vi "KH TURCK ETHERNETIP Init.vi"(6 "EIP_DO":T1 {"Nr" max=63; "Chan" max=63}, 7 "EIP_DI":T3={"Signal Name"=["IOL0", "IOL2", "ARFID0", "ARFID1", "BRFID2", "BRFID3", "ADXP1", "ADXP3", "ADXP4", "ADXP5", "BDXP0", "BDXP4", "BDXP5", "BDXP6"], "Description"=[], "Chan"=[], "Inv"=[], "Nr"=[1, 1, 1, 1, 2, 2, 1, 1, 1, 1, 2, 2, 2, 2], "SensorType"=[enum."TBEN-S2-4IOL", enum."TBEN-S2-4IOL", enum."TBEN-S2-2RFID-4DXP", enum."TBEN-S2-2RFID-4DXP", enum."TBEN-S2-2RFID-4DXP", enum."TBEN-S2-2RFID-4DXP", enum."TBEN-S1-8DXP", enum."TBEN-S1-8DXP", enum."TBEN-S1-8DXP", enum."TBEN-S1-8DXP", enum."TBEN-S1-8DXP", enum."TBEN-S1-8DXP", enum."TBEN-S1-8DXP", enum."TBEN-S1-8DXP"]} {"Nr" max=63; "Chan" max=63}, 8 "err in":errorcluster caption="error", 9 "TimeoutRFID":dbl=5.0 format="%#_13g", 10 "Parameter RFID Array":T4(array[cluster])=[{"NumberOfBytes0"=312, "SizeFragmentRead1"=128, "SizeFragmentRead0"=128, "SizeFragmentWrite0"=128, "SizeFragmentWrite1"=128, "NumberOfBytes1"=312}, {"NumberOfBytes0"=312, "SizeFragmentRead1"=128, "SizeFragmentRead0"=128, "SizeFragmentWrite0"=128, "SizeFragmentWrite1"=128, "NumberOfBytes1"=312}]) -> (0 "err out":errorcluster caption="error")   [LabVIEW 2021]
uses:
  KH_DAQ 17.04/Turck/KH_DAQ_TURCK_TypeDefs_Cluster DI.ctl
  KH EthernetIPConfig 17.14/KH EthernetIPConfig TypeDefs ModuleTyp.ctl
  KH_DAQ 17.04/Turck/KH_DAQ_TURCK_TypeDefs_Cluster DO.ctl
  KH TURCK ETHERNETIP TDef Enum IOL Data.ctl
  KH TURCK ETHERNETIP TDefCluster TBEN-S2-2RFID-4DXP Input Values.ctl
  KH EthernetIP 17.19/KH_EthernetIP_Globals.vi
  KH TURCK ETHERNETIP Global.vi
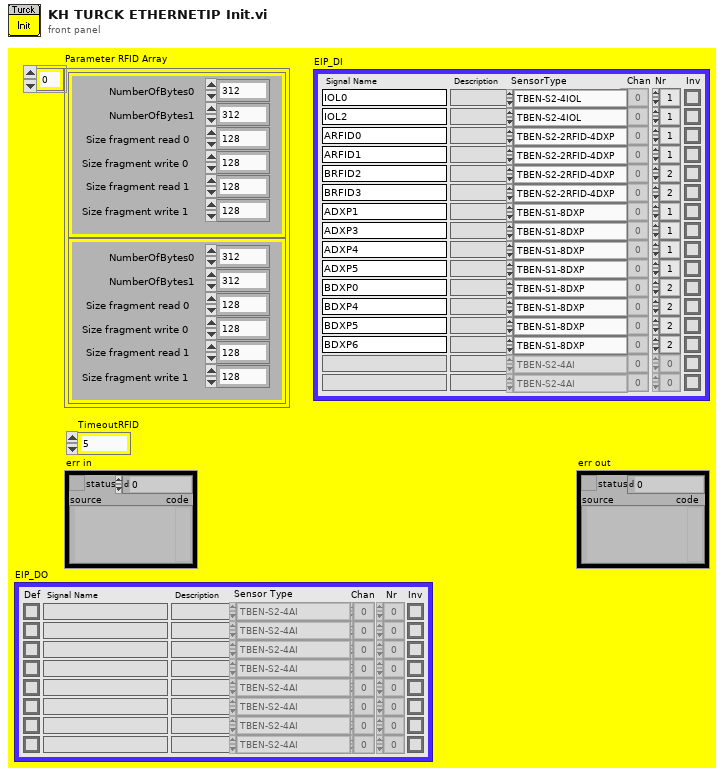
[diagram p1: front panel]
types:
  T1 = typedef "KH_DAQ_TURCK_TypeDefs_Cluster DO.ctl" = cluster{"Def":bool[], "Signal Name":string[], "Description":string[], "Chan":u16[], "Inv":bool[], "Nr":u16[], "SensorType":T2[]}
  T2 = typedef "KH EthernetIPConfig TypeDefs ModuleTyp.ctl" = enum16{"TBEN-S2-4AI", "TBEN-S1-8DXP", "TBEN-S2-2RFID-4DXP", "TBEN-S2-4AO", "TBEN-S2-4IOL"}
  T3 = typedef "KH_DAQ_TURCK_TypeDefs_Cluster DI.ctl" = cluster{"Signal Name":string[], "Description":string[], "Chan":u16[], "Inv":bool[], "Nr":u16[], "SensorType":T2[]}
  T4 = cluster{"NumberOfBytes0":i32, "SizeFragmentRead1":i32, "SizeFragmentRead0":i32, "SizeFragmentWrite0":i32, "SizeFragmentWrite1":i32, "NumberOfBytes1":i32}[]
  T5 = cluster{"Data":bool[], "Overcurrent":bool[], "Overcurrent VAUX1 Ch0-3":bool, "Overcurrent VAUX2 Ch4-7":bool, "Latch Input":bool[], "Counter value":u32, "Counter frequency (Hz)":u16, "Status":u8, "Overcurrent PWM Output 3":u8, "Overcurrent PWM Output 7":u8, "Module Diagnostics Available":bool, "INFO: ARGEE Project Running":bool, "Undervoltage V2":bool, "Undervoltage V1":bool, "Force Mode Enabled":bool}
  T6 = cluster{"Overload Ch0":bool, "Overload Ch1":bool, "Overload Ch2":bool, "Overload Ch3":bool, "Wirebreak Ch0":bool, "Wirebreak Ch1":bool, "Wirebreak Ch2":bool, "Wirebreak Ch3":bool, "Module Diagnostics Available":bool, "INFO: ARGEE Project Running":bool, "Undervoltage V2":bool, "Undervoltage V1":bool, "Internal Error":bool, "Force Mode Enabled":bool}
  T7 = cluster{"Data":i16[], "upper Limit CH0":bool, "upper Limit CH1":bool, "upper Limit CH2":bool, "upper Limit CH3":bool, "Overflow CH0":bool, "Overflow CH1":bool, "Overflow CH2":bool, "Overflow CH3":bool, "Underflow CH0":bool, "Underflow CH1":bool, "Underflow CH2":bool, "Underflow CH3":bool, "CJC Wire Break CH0":bool, "CJC Wire Break CH1":bool, "CJC Wire Break CH2":bool, "CJC Wire Break CH3":bool, "Overcurrent (RTD) CH0":bool, "Overcurrent (RTD) CH1":bool, "Overcurrent (RTD) CH2":bool, "Overcurrent (RTD) CH3":bool, "Wire Break CH0":bool, "Wire Break CH1":bool, "Wire Break CH2":bool, "Wire Break CH3":bool, "Overcurrent supply VAUX1 CH0":bool, "Overcurrent supply VAUX1 CH1":bool, "Overcurrent supply VAUX1 CH2":bool, "Overcurrent supply VAUX1 CH3":bool, "Lower limit value underrun CH0":bool, "Lower limit value underrun CH1":bool, "Lower limit value underrun CH2":bool, "Lower limit value underrun CH3":bool, "Module Diagnostics Available":bool, "INFO: ARGEE Project Running":bool, "Undervoltage Field Supply V2":bool, "Undervoltage Field Supply V1":bool, "Internal Error":bool, "Force Mode Enabled":bool}
  T8 = typedef "KH TURCK ETHERNETIP TDefCluster TBEN-S2-2RFID-4DXP Input Values.ctl" = cluster{"Station Status Word (Input Data Mapping)":cluster{"Module diagnostics avaliable":bool, "INFO: ARGEE Project Running":bool, "Undervoltage V2":bool, "Undervoltage V1":bool, "Internal Error":bool, "I/O-ASSISTANT Force Mode active":bool}, "RFID control/status 0 (Input Data Mapping)":cluster{"Tag present at r/w head":bool[], "response code":u16, "loop counter":u8, "Length":u16, "Error code":u16, "Tag counter":u16, "Data (Bytes) available":u16, "Read fragment No.":u8, "Write fragment No.":u8, "Tag present at r/w head bit":bool, "HF r/w head switched on":bool, "Continuous mode active":bool, "Antenna detuned at HF read/write head":bool, "Parameter not supported by read/write head":bool, "Error reported by read/write head":bool, "Not connected to read/write head":bool}, "RFID read data 0 (Input Data Mapping)":u8[], "RFID control/status 1 (Input Data Mapping)":cluster{"response code":u16, "Loop counter":u8, "Length":u16, "Error code":u16, "Tag counter":u16, "Data (Bytes) available":u16, "Read fragment No.":u8, "Write fragment No.":u8, "Tag present at r/w head bit":bool, "HF r/w head switched on":bool, "Continuous mode active":bool, "Antenna detuned at HF read/write head":bool, "Parameter not supported by read/write head":bool, "Error reported by read/write head":bool, "Not connected to read/write head":bool, "Tag present at r/w head":bool[]}, "RFID read data 1 (Input Data Mapping)":u8[], "RFID diagnostics (Input Data Mapping)":cluster{"Overcurrent supply VAUX1 (a)":bool, "Parameterization error (a)":bool, "Configuration via DTM active (a)":bool, "Buffer full (a)":bool, "Antenna detuned at HF read/write head (a)":bool[], "Parameter not supported by read/write head (a)":bool[], "Error reported by read/write head (a)":bool[], "Not connected to read/write head (a)":bool[], "Overcurrent supply VAUX1 (b)":bool, "Parameterization error (b)":bool, "Configuration via DTM active (b)":bool, "Buffer full (b)":bool, "Antenna detuned at HF read/write head (b)":bool[], "Parameter not supported by read/write head (b)":bool[], "Error reported by read/write head (b)":bool[], "Not connected to read/write head (b)":bool[]}, "DXP diagnostics (Input Data Mapping)":cluster{"Overcurrent VAUX2 Ch4/5":bool, "Overcurrent VAUX2 Ch6/7":bool, "Channel 4 - Output overcurrent":bool, "Channel 5 - Output overcurrent":bool, "Channel 6 - Output overcurrent":bool, "Channel 7 - Output overcurrent":bool}, "DXP (Input Data Mapping)":cluster{"Channel 4 - Input value":bool, "Channel 5 - Input value":bool, "Channel 6 - Input value":bool, "Channel 7 - Input value":bool}}
  T9 = typedef "KH TURCK ETHERNETIP TDef Enum IOL Data.ctl" = cluster{"Data_Port1":u16[], "Data_Port3":u16[], "Data_Port5":u16[], "Data_Port7":u16[], "Status":cluster{"Undervoltage Field Supply V2":bool, "Overvoltage Field Supply V1":bool, "Undervoltage Field Supply V1":bool, "Internal Error":bool, "Module Diagnostics Available":bool, "Station Configuration Changed":bool, "Overcurrent Isys":bool, "Overvoltage Field Supply V2":bool, "Force Mode Enabled":bool}, "Diagnostics":cluster{"Channel 2 - Output signal overcurrent":bool, "Channel 4 - Output signal overcurrent":bool, "Channel 6 - Output signal overcurrent":bool, "Channel 8 - Output signal overcurrent":bool, "Channel 1 - Wrong or missing device":bool, "Channel 3 - Wrong or missing device":bool, "Channel 5 - Wrong or missing device":bool, "Channel 7 - Wrong or missing device":bool, "Channel 1 - Data storage error":bool, "Channel 3 - Data storage error":bool, "Channel 5 - Data storage error":bool, "Channel 7 - Data storage error":bool, "Channel 1 - Process input data invalid":bool, "Channel 3 - Process input data invalid":bool, "Channel 5 - Process input data invalid":bool, "Channel 7 - Process input data invalid":bool, "Channel 1 - Hardware error":bool, "Channel 3 - Hardware error":bool, "Channel 5 - Hardware error":bool, "Channel 7 - Hardware error":bool, "Channel 1 - Maintenance events":bool, "Channel 3 - Maintenance events":bool, "Channel 5 - Maintenance events":bool, "Channel 7 - Maintenance events":bool, "Channel 1 - Out of spec. error":bool, "Channel 3 - Out of spec. error":bool, "Channel 5 - Out of spec. error":bool, "Channel 7 - Out of spec. error":bool, "Channel 1 - Parameterization error":bool, "Channel 3 - Parameterization error":bool, "Channel 5 - Parameterization error":bool, "Channel 1 - Overtemperature":bool, "Channel 3 - Overtemperature":bool, "Channel 5 - Overtemperature":bool, "Channel 7 - Overtemperature":bool, "Channel 1 - Lower limit value underrun":bool, "Channel 3 - Lower limit value underrun":bool, "Channel 5 - Lower limit value underrun":bool, "Channel 7 - Lower limit value underrun":bool, "Channel 1 - Upper limit value exceeded":bool, "Channel 3 - Upper limit value exceeded":bool, "Channel 5 - Upper limit value exceeded":bool, "Channel 7 - Upper limit value exceeded":bool, "Channel 1 - Undervoltage":bool, "Channel 3 - Undervoltage":bool, "Channel 5 - Undervoltage":bool, "Channel 7 - Undervoltage":bool, "Channel 1 - Overvoltage":bool, "Channel 3 - Overvoltage":bool, "Channel 5 - Overvoltage":bool, "Channel 7 - Overvoltage":bool, "Channel 1 - Overload":bool, "Channel 3 - Overload":bool, "Channel 5 - Overload":bool, "Channel 7 - Overload":bool, "Channel 1 - Common error":bool, "Channel 3 - Common error":bool, "Channel 5 - Common error":bool, "Channel 7 - Common error":bool, "Channel 1 - Port parameterization error":bool, "Channel 3 - Port parameterization error":bool, "Channel 5 - Port parameterization error":bool, "Channel 7 - Parameterization error":bool, "Channel 7 - Port parameterization error":bool}, "Events":cluster{"Event":u8[], "Qualifier":u8[], " Event code":u16[]}, "DXP":cluster{"DI Input value 2":bool, "DI Input value 4":bool, "DI Input value 6":bool, "DI Input value 8":bool, "DI Input 1":bool, "DI Input 3":bool, "DI Input 5":bool, "DI Input 7":bool, "Input values valid 1":bool, "Input values valid 3":bool, "Input values valid 5":bool, "Input values valid 7":bool}}
  T10 = typedef "KH EthernetIPConfig TDef Config.ctl" = cluster{"Typ":T2, "Name":string, "Nr.":i32, "InputOutput":enum16{"Input", "Output"}[]}
  T11 = cluster{"Data":i16[], "upper Limit CH0":bool, "upper Limit CH1":bool, "upper Limit CH2":bool, "upper Limit CH3":bool, "Overflow CH0":bool, "Overflow CH1":bool, "Overflow CH2":bool, "Overflow CH3":bool, "Underflow CH0":bool, "Underflow CH1":bool, "Underflow CH2":bool, "Underflow CH3":bool, "CJC Wire Break CH0":bool, "CJC Wire Break CH1":bool, "CJC Wire Break CH2":bool, "CJC Wire Break CH3":bool, "Overcurrent (RTD) CH0":bool, "Overcurrent (RTD) CH1":bool, "Overcurrent (RTD) CH2":bool, "Overcurrent (RTD) CH3":bool, "Wire Break CH0":bool, "Wire Break CH1":bool, "Wire Break CH2":bool, "Wire Break CH3":bool, "Overcurrent supply VAUX1 CH0":bool, "Overcurrent supply VAUX1 CH1":bool, "Overcurrent supply VAUX1 CH2":bool, "Overcurrent supply VAUX1 CH3":bool, "Lower limit value underrun CH0":bool, "Lower limit value underrun CH1":bool, "Lower limit value underrun CH2":bool, "Lower limit value underrun CH3":bool, "Module Diagnostics Available":bool, "INFO: ARGEE Project Running":bool, "Undervoltage Field Supply V2":bool, "Undervoltage Field Supply V1":bool, "Internal Error":bool, "Force Mode Enabled":bool}[]
  T12 = cluster{"Overload Ch0":bool, "Overload Ch1":bool, "Overload Ch2":bool, "Overload Ch3":bool, "Wirebreak Ch0":bool, "Wirebreak Ch1":bool, "Wirebreak Ch2":bool, "Wirebreak Ch3":bool, "Module Diagnostics Available":bool, "INFO: ARGEE Project Running":bool, "Undervoltage V2":bool, "Undervoltage V1":bool, "Internal Error":bool, "Force Mode Enabled":bool}[]
  T13 = cluster{"Data":bool[], "Overcurrent":bool[], "Overcurrent VAUX1 Ch0-3":bool, "Overcurrent VAUX2 Ch4-7":bool, "Latch Input":bool[], "Counter value":u32, "Counter frequency (Hz)":u16, "Status":u8, "Overcurrent PWM Output 3":u8, "Overcurrent PWM Output 7":u8, "Module Diagnostics Available":bool, "INFO: ARGEE Project Running":bool, "Undervoltage V2":bool, "Undervoltage V1":bool, "Force Mode Enabled":bool}[]
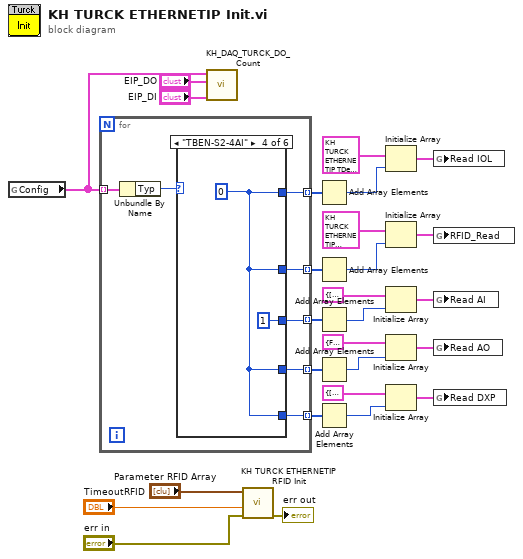
[diagram p0: block diagram]
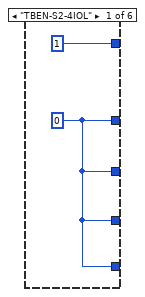
[diagram p2: hidden frame]
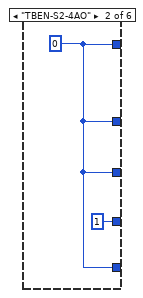
[diagram p3: hidden frame]
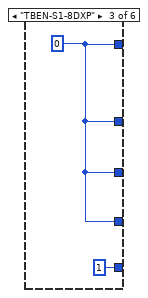
[diagram p4: hidden frame]
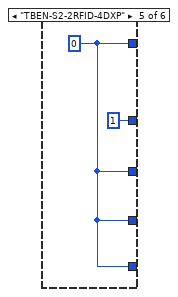
[diagram p5: hidden frame]
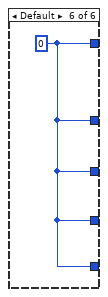
[diagram p6: hidden frame]
diagram:
  n1 = global read "KH_EthernetIP_Globals.vi" "Config"() -> (w2:T10[])
  n2 = for {
    tunnel: w2 -> [w34] mode=indexing
    tunnel: [w32] -> w27 mode=indexing
    tunnel: [w31] -> w20 mode=indexing
    tunnel: [w30] -> w19 mode=indexing
    tunnel: [w29] -> w18 mode=indexing
    tunnel: [w28] -> w17 mode=indexing
    n3 = Unbundle By Name(w34) -> ("Typ"=w33:T2)
    n4 = case shown="\"TBEN-S2-4AI\"" w33 {
      tunnel: [1 w37 w40 w42 w44 w45] -> w32
      tunnel: [w35 w37 w40 w42 1 w45] -> w31
      tunnel: [w35 w37 w40 1 w44 w45] -> w30
      tunnel: [w35 1 w40 w42 w44 w45] -> w29
      tunnel: [w35 w37 1 w42 w44 w45] -> w28
      frame "TBEN-S2-4IOL" {
        w35 = 0
      }
      frame "TBEN-S2-4AO" {
        w37 = 0
      }
      frame "TBEN-S1-8DXP" {
        w40 = 0
      }
      frame "TBEN-S2-4AI" {
        w42 = 0
      }
      frame "TBEN-S2-2RFID-4DXP" {
        w44 = 0
      }
      frame Default {
        w45 = 0
      }
    }
  }
  n5 = call "KH_DAQ_TURCK_DO_Count.vi"("EIP_DI"="EIP_DI", "EIP_DO"="EIP_DO", "Config"=w2) -> ()  [unwired: 9 in]
  n6 = call "KH TURCK ETHERNETIP RFID Init.vi"("err in"="err in", "Timeout"="TimeoutRFID", "Parameter RFID Array"="Parameter RFID Array") -> ("err out"=→"err out":errorcluster)  [unwired: 8 in]
  n7 = Add Array Elements(numeric array=w27) -> (sum=w25:i32)
  n8 = Add Array Elements(numeric array=w20) -> (sum=w16:i32)
  n9 = Add Array Elements(numeric array=w19) -> (sum=w15:i32)
  n10 = Add Array Elements(numeric array=w18) -> (sum=w14:i32)
  n11 = Add Array Elements(numeric array=w17) -> (sum=w13:i32)
  n12 = Initialize Array(T9 {"Data_Port1"=[], "Data_Port3"=[], "Data_Port5"=[], "Data_Port7"=[], "Status"={"Undervoltage Field Supply V2"=FALSE, "Overvoltage Field Supply V1"=FALSE, "Undervoltage Field Supply V1"=FALSE, "Internal Error"=FALSE, "Module Diagnostics Available"=FALSE, "Station Configuration Changed"=FALSE, "Overcurrent Isys"=FALSE, "Overvoltage Field Supply V2"=FALSE, "Force Mode Enabled"=FALSE}, "Diagnostics"={"Channel 2 - Output signal overcurrent"=FALSE, "Channel 4 - Output signal overcurrent"=FALSE, "Channel 6 - Output signal overcurrent"=FALSE, "Channel 8 - Output signal overcurrent"=FALSE, "Channel 1 - Wrong or missing device"=FALSE, "Channel 3 - Wrong or missing device"=FALSE, "Channel 5 - Wrong or missing device"=FALSE, "Channel 7 - Wrong or missing device"=FALSE, "Channel 1 - Data storage error"=FALSE, "Channel 3 - Data storage error"=FALSE, "Channel 5 - Data storage error"=FALSE, "Channel 7 - Data storage error"=FALSE, "Channel 1 - Process input data invalid"=FALSE, "Channel 3 - Process input data invalid"=FALSE, "Channel 5 - Process input data invalid"=FALSE, "Channel 7 - Process input data invalid"=FALSE, "Channel 1 - Hardware error"=FALSE, "Channel 3 - Hardware error"=FALSE, "Channel 5 - Hardware error"=FALSE, "Channel 7 - Hardware error"=FALSE, "Channel 1 - Maintenance events"=FALSE, "Channel 3 - Maintenance events"=FALSE, "Channel 5 - Maintenance events"=FALSE, "Channel 7 - Maintenance events"=FALSE, "Channel 1 - Out of spec. error"=FALSE, "Channel 3 - Out of spec. error"=FALSE, "Channel 5 - Out of spec. error"=FALSE, "Channel 7 - Out of spec. error"=FALSE, "Channel 1 - Parameterization error"=FALSE, "Channel 3 - Parameterization error"=FALSE, "Channel 5 - Parameterization error"=FALSE, "Channel 1 - Overtemperature"=FALSE, "Channel 3 - Overtemperature"=FALSE, "Channel 5 - Overtemperature"=FALSE, "Channel 7 - Overtemperature"=FALSE, "Channel 1 - Lower limit value underrun"=FALSE, "Channel 3 - Lower limit value underrun"=FALSE, "Channel 5 - Lower limit value underrun"=FALSE, "Channel 7 - Lower limit value underrun"=FALSE, "Channel 1 - Upper limit value exceeded"=FALSE, "Channel 3 - Upper limit value exceeded"=FALSE, "Channel 5 - Upper limit value exceeded"=FALSE, "Channel 7 - Upper limit value exceeded"=FALSE, "Channel 1 - Undervoltage"=FALSE, "Channel 3 - Undervoltage"=FALSE, "Channel 5 - Undervoltage"=FALSE, "Channel 7 - Undervoltage"=FALSE, "Channel 1 - Overvoltage"=FALSE, "Channel 3 - Overvoltage"=FALSE, "Channel 5 - Overvoltage"=FALSE, "Channel 7 - Overvoltage"=FALSE, "Channel 1 - Overload"=FALSE, "Channel 3 - Overload"=FALSE, "Channel 5 - Overload"=FALSE, "Channel 7 - Overload"=FALSE, "Channel 1 - Common error"=FALSE, "Channel 3 - Common error"=FALSE, "Channel 5 - Common error"=FALSE, "Channel 7 - Common error"=FALSE, "Channel 1 - Port parameterization error"=FALSE, "Channel 3 - Port parameterization error"=FALSE, "Channel 5 - Port parameterization error"=FALSE, "Channel 7 - Parameterization error"=FALSE, "Channel 7 - Port parameterization error"=FALSE}, "Events"={"Event"=[], "Qualifier"=[], " Event code"=[]}, "DXP"={"DI Input value 2"=FALSE, "DI Input value 4"=FALSE, "DI Input value 6"=FALSE, "DI Input value 8"=FALSE, "DI Input 1"=FALSE, "DI Input 3"=FALSE, "DI Input 5"=FALSE, "DI Input 7"=FALSE, "Input values valid 1"=FALSE, "Input values valid 3"=FALSE, "Input values valid 5"=FALSE, "Input values valid 7"=FALSE}} ("Data_IOL"), w25) -> (w8:T9[])
  n13 = Initialize Array(T8 {"Station Status Word (Input Data Mapping)"={"Module diagnostics avaliable"=FALSE, "INFO: ARGEE Project Running"=FALSE, "Undervoltage V2"=FALSE, "Undervoltage V1"=FALSE, "Internal Error"=FALSE, "I/O-ASSISTANT Force Mode active"=FALSE}, "RFID control/status 0 (Input Data Mapping)"={"Tag present at r/w head"=[], "response code"=0, "loop counter"=0, "Length"=0, "Error code"=0, "Tag counter"=0, "Data (Bytes) available"=0, "Read fragment No."=0, "Write fragment No."=0, "Tag present at r/w head bit"=FALSE, "HF r/w head switched on"=FALSE, "Continuous mode active"=FALSE, "Antenna detuned at HF read/write head"=FALSE, "Parameter not supported by read/write head"=FALSE, "Error reported by read/write head"=FALSE, "Not connected to read/write head"=FALSE}, "RFID read data 0 (Input Data Mapping)"=[], "RFID control/status 1 (Input Data Mapping)"={"response code"=0, "Loop counter"=0, "Length"=0, "Error code"=0, "Tag counter"=0, "Data (Bytes) available"=0, "Read fragment No."=0, "Write fragment No."=0, "Tag present at r/w head bit"=FALSE, "HF r/w head switched on"=FALSE, "Continuous mode active"=FALSE, "Antenna detuned at HF read/write head"=FALSE, "Parameter not supported by read/write head"=FALSE, "Error reported by read/write head"=FALSE, "Not connected to read/write head"=FALSE, "Tag present at r/w head"=[]}, "RFID read data 1 (Input Data Mapping)"=[], "RFID diagnostics (Input Data Mapping)"={"Overcurrent supply VAUX1 (a)"=FALSE, "Parameterization error (a)"=FALSE, "Configuration via DTM active (a)"=FALSE, "Buffer full (a)"=FALSE, "Antenna detuned at HF read/write head (a)"=[], "Parameter not supported by read/write head (a)"=[], "Error reported by read/write head (a)"=[], "Not connected to read/write head (a)"=[], "Overcurrent supply VAUX1 (b)"=FALSE, "Parameterization error (b)"=FALSE, "Configuration via DTM active (b)"=FALSE, "Buffer full (b)"=FALSE, "Antenna detuned at HF read/write head (b)"=[], "Parameter not supported by read/write head (b)"=[], "Error reported by read/write head (b)"=[], "Not connected to read/write head (b)"=[]}, "DXP diagnostics (Input Data Mapping)"={"Overcurrent VAUX2 Ch4/5"=FALSE, "Overcurrent VAUX2 Ch6/7"=FALSE, "Channel 4 - Output overcurrent"=FALSE, "Channel 5 - Output overcurrent"=FALSE, "Channel 6 - Output overcurrent"=FALSE, "Channel 7 - Output overcurrent"=FALSE}, "DXP (Input Data Mapping)"={"Channel 4 - Input value"=FALSE, "Channel 5 - Input value"=FALSE, "Channel 6 - Input value"=FALSE, "Channel 7 - Input value"=FALSE}} ("element"), w16) -> (w10:T8[])
  n14 = Initialize Array(T7 {"Data"=[], "upper Limit CH0"=FALSE, "upper Limit CH1"=FALSE, "upper Limit CH2"=FALSE, "upper Limit CH3"=FALSE, "Overflow CH0"=FALSE, "Overflow CH1"=FALSE, "Overflow CH2"=FALSE, "Overflow CH3"=FALSE, "Underflow CH0"=FALSE, "Underflow CH1"=FALSE, "Underflow CH2"=FALSE, "Underflow CH3"=FALSE, "CJC Wire Break CH0"=FALSE, "CJC Wire Break CH1"=FALSE, "CJC Wire Break CH2"=FALSE, "CJC Wire Break CH3"=FALSE, "Overcurrent (RTD) CH0"=FALSE, "Overcurrent (RTD) CH1"=FALSE, "Overcurrent (RTD) CH2"=FALSE, "Overcurrent (RTD) CH3"=FALSE, "Wire Break CH0"=FALSE, "Wire Break CH1"=FALSE, "Wire Break CH2"=FALSE, "Wire Break CH3"=FALSE, "Overcurrent supply VAUX1 CH0"=FALSE, "Overcurrent supply VAUX1 CH1"=FALSE, "Overcurrent supply VAUX1 CH2"=FALSE, "Overcurrent supply VAUX1 CH3"=FALSE, "Lower limit value underrun CH0"=FALSE, "Lower limit value underrun CH1"=FALSE, "Lower limit value underrun CH2"=FALSE, "Lower limit value underrun CH3"=FALSE, "Module Diagnostics Available"=FALSE, "INFO: ARGEE Project Running"=FALSE, "Undervoltage Field Supply V2"=FALSE, "Undervoltage Field Supply V1"=FALSE, "Internal Error"=FALSE, "Force Mode Enabled"=FALSE} ("TBEN-S2-4AI Input Values"), w15) -> (w12:T11)
  n15 = Initialize Array(T6 {"Overload Ch0"=FALSE, "Overload Ch1"=FALSE, "Overload Ch2"=FALSE, "Overload Ch3"=FALSE, "Wirebreak Ch0"=FALSE, "Wirebreak Ch1"=FALSE, "Wirebreak Ch2"=FALSE, "Wirebreak Ch3"=FALSE, "Module Diagnostics Available"=FALSE, "INFO: ARGEE Project Running"=FALSE, "Undervoltage V2"=FALSE, "Undervoltage V1"=FALSE, "Internal Error"=FALSE, "Force Mode Enabled"=FALSE} ("TBEN-S2-4AO Input Values"), w14) -> (w9:T12)
  n16 = Initialize Array(T5 {"Data"=[], "Overcurrent"=[], "Overcurrent VAUX1 Ch0-3"=FALSE, "Overcurrent VAUX2 Ch4-7"=FALSE, "Latch Input"=[], "Counter value"=0, "Counter frequency (Hz)"=0, "Status"=0, "Overcurrent PWM Output 3"=0, "Overcurrent PWM Output 7"=0, "Module Diagnostics Available"=FALSE, "INFO: ARGEE Project Running"=FALSE, "Undervoltage V2"=FALSE, "Undervoltage V1"=FALSE, "Force Mode Enabled"=FALSE} ("TBEN-S1-8DXP Input Values"), w13) -> (w11:T13)
  n17 = global write "KH TURCK ETHERNETIP Global.vi" "Read IOL"(w8) -> ()
  n18 = global write "KH TURCK ETHERNETIP Global.vi" "RFID_Read"(w10) -> ()
  n19 = global write "KH TURCK ETHERNETIP Global.vi" "Read AI"(w12) -> ()
  n20 = global write "KH TURCK ETHERNETIP Global.vi" "Read AO"(w9) -> ()
  n21 = global write "KH TURCK ETHERNETIP Global.vi" "Read DXP"(w11) -> ()
